vi "EventLog.Filter.vi"(0 "data in":T3[](array[typedef]) {"ts" format="%<%X\n%x>T"}, 1 "Event.Sets":T1 {"Source" items=["Scanner Prod"]; "Level" items=["Warning"]; "dtm_End" format="%<%.1X\n%x>T"; "dtm_Begin" format="%<%.1X\n%x>T"}) -> (2 "data out":T3[](array[typedef]) {"ts" format="%<%X\n%x>T"})   [LabVIEW 2016]
uses:
  EventLog.EventGui.ctl
  EventLog.EventLevel.ctl
  EventLog.EventSource.ctl
  Translator/Translator.Message.ctl
  EventLog.Gui.Sets.ctl
  EventLog.EventLevelOperatorGui.ctl
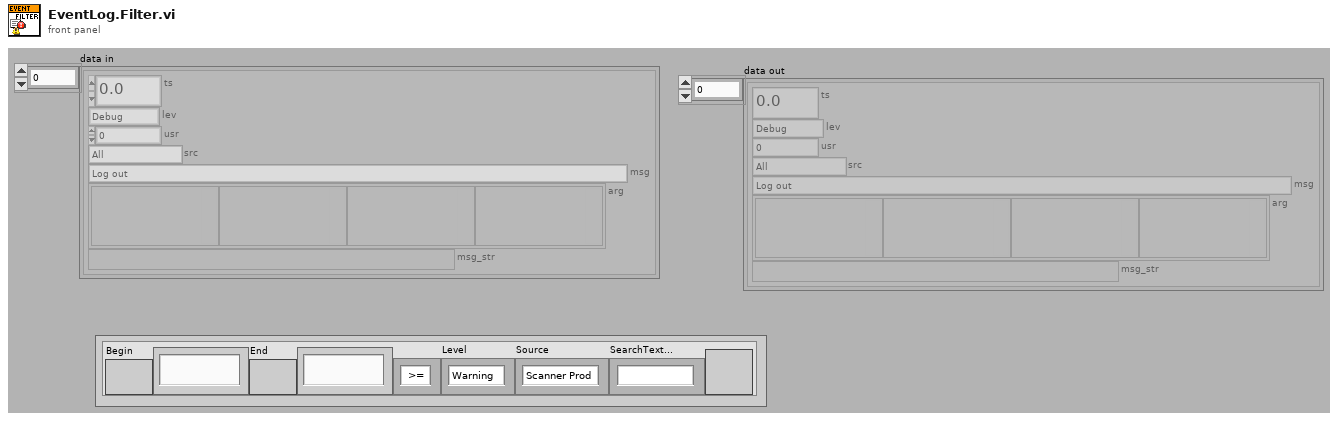
[diagram p1: front panel]
types:
  T1 = typedef "EventLog.Gui.Sets.ctl" = cluster{"IncludeBegin":bool, "dtm_Begin":timestamp, "IncludeEnd":bool, "dtm_End":timestamp, "Events Level Operator":T2, "Level":u16, "Source":u16, "SearchText":string, "Freeze":bool}
  T2 = typedef "EventLog.EventLevelOperatorGui.ctl" = enum16{">=", "=", "<="}
  T3 = typedef "EventLog.EventGui.ctl" = cluster{"ts":dbl, "lev":T4, "usr":i32, "src":T5, "msg":T6, "arg":variant[], "msg_str":string}
  T4 = typedef "EventLog.EventLevel.ctl" = enum8{"Debug", "Info", "Warning", "Error"}
  T5 = typedef "EventLog.EventSource.ctl" = enum16{"All", "Gui", "Ref", "File", "Arch", "Seq", "CPX", "DB", "Laser", "Scan.P", "Scan.O"}
  T6 = typedef "Translator.Message.ctl" = enum16{"-", "Event confirmed", "Log out", "Log in", "Shutdown", "Cancel", "Start", "Begin time", "End time", "Duration", "Service Mode", "Ignore Results", "Serial Format", "On", "Off", "OK", "NOK", "NOK %s", "Home", "Work", "Close", "Open", "In progress...", "Missing", "Empty", "Hardware failure", "Initial", "Default", "Total", "Out of range", "Free disk space is below 1GB - contact technician", "Error %d >> %s", "Error %d >> %s >> %s", "Msg %d >> %s", "Laser msg %d %s", "Laser cmd error %s %d", "Laser cmd failed %s", "Laser cmd warning %s", "Laser disconnected", "Laser status %s", "Laser already started", "Laser job unkonwn %s", "Laser job missing %s", "Laser job select failure %s", "Unable to start laser printing (%s)", "Unable to stop laser printing (%s)", "Laser marking aborted", "Laser marking timeout", "Unable to reset Laser Interlock (%s)", "Unable to trigger Laser. Laser not ready (%s)", "Laser job '%s' coordinates not configured", "Starting %s", "Quitting %s", "Configured", "Initializing", "Quitting", "Loading", "Loaded %d results", "Loaded %d events", "Running", "Stopped", "Summary", "Laser", "Do you want to continue?", "Do you want to delete the configuration?", "The configuration is being used by an order. Unable to delete!", "Press confirm button", "Station is not based. Do you want to exit?", "Station requires changeover. Do you want to run the test?", "Test options are not set as default. Do you want to continue?", "Formatting of WabcoNo is disabled. Do you want to continue?", "Product not detected. Do you want to continue?", "Product scan failed. Do you want to continue?", "Calibration", "Log out?", "System", "All", "IDLE", "Translating...%s", "Not found", "Alarm %s", "Run", "Skip", "Abort", "Repeat", "Please wait...", "Database disconnected", "Database disconnected - changeover disabled!", "Login to database successful", "Login to database failed: %d; %s", "Unable to check the product status of reference %d - database disconnected", "Unable to set the product status of reference %d - database disconnected", "Variant file backup %s", "Read variant (%s)", "Result", "Station armed!", "Station requires changeover!", "Select reference number...", "EMERGENCY BUTTON - press Control button", "EMERGENCY DOOR - press Control button", "Resetting Emergency...", "Unable to reset safety circuit - Emergency Button pressed", "Unable to reset safety circuit - Emergency Side Door open", "Station not based", "Station based", "Station not empty", "Station basing...", "No order", "Press Start to begin new order", "Scanning new order", "Order NOK. Correct or scan again", "Order OK. Press Accept", "Order ready", "Revolver incorrect", "Fork incorrect", "Revolver missing", "Revolver empty", "Container missing", "Offline results", "Offline statistics", "Updating statistics %.1f %%", "DMC Configurator", "Door open", "Close the front door", "Press start button", "Done. Open the front door", "Running...", "Running...%.1f %%", "Pause %s", "Pause %s. NOK container missing", "Pause %s. OK container missing", "Pause %s. Revolver empty", "Pause %s. Revolver missing", "Pause %s. Revolver incorrect", "Pause %s. Fork missing", "Pause %s. Fork incorrect", "Pause %s. Too many failures", "Pause %s. Unloading failure", "Pause %s. One slot is not working", "Pause %s. Part order is done. Empty OK container", "Pause %s. Unable to move product to slot", "Pause %s. Unable to move back product pusher", "Pause %s. Unable to lift product", "Pause %s. Unable to move back product lifter", "Pause %s. Unable to move product arm to Work", "Pause %s. Unable to move product arm to NOK", "Pause %s. Unable to move product arm to OK", "Pause %s. Unable to unsuck the NOK product", "Pause %s. Unable to drop the NOK product", "Pause %s. Product OK missing", "Pause %s. Unable to unsuck the OK product", "Pause %s. Unable to drop the OK product", "Stopping...", "File '%s' is missing", "File '%s' is broken", "File '%s' is running", "Log file started (%s)", "Log file ended (%s)", "Log file stopped (%s)", "Log file ignored (%s)", "Log file exported (%s)", "Log file export failed (%s)", "Wrong serial number in log file", "Wrong reference number in log file", "Test steps are missing", "%s = %.3f", "Process param '%s' not found in DB", "Process param '%s' wrong order", "Process param '%s' value %.3f out of limits (%.3f; %.3f)", "Step%d param '%s' not found in DB", "Step%d param '%s' wrong order", "Step%d param '%s' value %.3f out of limits (%.3f; %.3f)", "Step%d EV '%s' not found in DB", "Step%d EV '%s' wrong order", "\"%s\" not found in DB", "\"%s\" wrong order", "\"%s\" value %.3f out of limits (%.3f; %.3f)", "\"%s\" not found in software", "Process init (%s)", "Process started", "Process restarted", "Process run", "Process done", "Process done - remove OK container", "Process aborted", "Process aborted at work", "Process aborted at home", "Process error", "Process error at home", "Process error at work", "Process close", "Process pause", "Process continue", "Process door open", "Process door close", "Process pause at slot %s due to %s", "Select plate from the order to process", "Do you want to start the process?", "Do you want to continue the process?", "There is unfinished order. Do you want to put the new order?", "Product %s %d OK", "Product %s %d NOK", "Unable to unload the slot %s. Product missing in the slot", "Unable to unload the slot %s. Product already in the arm", "Unable to accept the product as OK. Product missing in slot %s", "Unable to accept the product as OK. Product could not drop into the container at slot %s", "Unable to accept the product as NOK. Product could not drop into the container at slot %s", "Scan failed. Error %s", "Scan failed. Scanner disconnected", "Scan failed. Wrong Wabco number %d, limit (%d,%d)", "Scan failed. Wrong serial number %d, limit (%d,%d)", "Scan failed. Wrong date %d, limit (%d,%d)", "Scan failed. Wrong product wabco number %d (expected %d)", "Scan failed. Wrong product serial number %d (expected > 0)", "Scan OK %s", "Scan failed. Unable to determine table position (%s)", "Scan failed. Timeout", "Tune failed. Scanner disconnected", "Tune failed. Timeout", "%s = %d", "%s = %d->%d", "Unable to set %s = %.2f - Air Pressure Inside off", "Unable to set digital output '%s' = %d", "Unable to activate air pressure inside - timeout", "Unable to activate air pressure inside - aborted", "Unable to switch on Air Main Valve - Air Pressure Inlet off", "Unable to switch on Air Main Valve - Door open", "Unable to switch off Air Main Valve - timeout", "Unable to switch off Air Main Valve - aborted", "Unable to rotate Table - timeout", "Unable to rotate Table - aborted", "Unable to rotate Table - Product Move not in Home position", "Unable to rotate Table - Air Pressure Inside off", "Unable to rotate Table - Product Lift A not in Home position", "Unable to rotate Table - Product Lift B not in Home position", "Unable to rotate Table - unlock before movement timeout", "Unable to rotate Table - lock after movement timeout", "Unable to move Table Lock to %s position - timeout", "Unable to move Table Lock to %s position - aborted", "Unable to move Table Lock to %s position - Air Pressure Inside off", "Unable to move Table Lock to %s position - Table not in position", "Unable to move Product Lift A to %s position - timeout", "Unable to move Product Lift B to %s position - timeout", "Unable to move Product Lift A to %s position - aborted", "Unable to move Product Lift B to %s position - aborted", "Unable to move Product Lift A to %s position - Air Pressure Inside off", "Unable to move Product Lift B to %s position - Air Pressure Inside off", "Unable to move Product Lift A to %s position - Table not locked", "Unable to move Product Lift B to %s position - Table not locked", "Unable to move Product Lift A to %s position - Product Arm not in Work position", "Unable to move Product Lift B to %s position - Product Arm not in Work position", "Unable to set Product Suction Gripper %s to %s - timeout", "Unable to set Product Suction Gripper %s to %s - aborted", "Unable to set Product Suction Gripper %s to %s - Air Pressure Inside off", "Unable to set Product Suction Gripper %s to %s - Table slot unkown", "Unable to move Product Arm to %s position - timeout", "Unable to move Product Arm to %s position - aborted", "Unable to move Product Arm to %s position - Air Pressure Inside off", "Unable to move Product Arm to %s position - Product Lift A not in Home position", "Unable to move Product Arm to %s position - Product Lift B not in Home position", "Unable to move Product to %s position - timeout", "Unable to move Product to %s position - aborted", "Unable to move Product to %s position - Air Pressure Inside off", "Unable to move Product to %s position - Table not in position"}
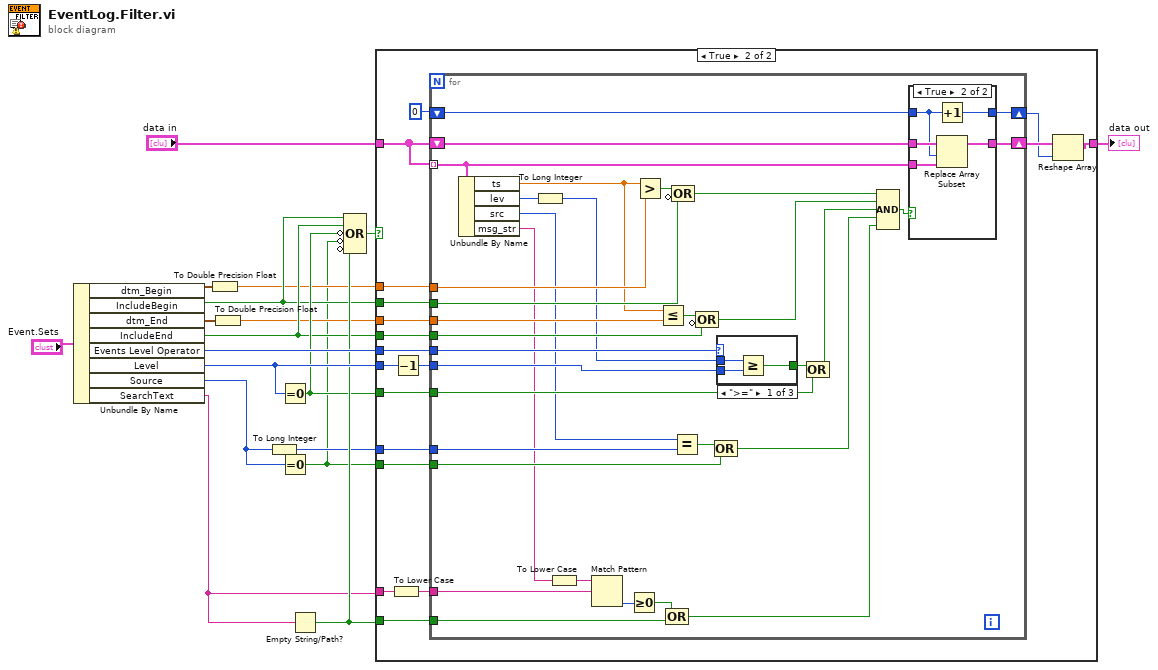
[diagram p0: block diagram]
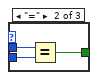
[diagram p4: hidden frame]
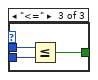
[diagram p5: hidden frame]
diagram:
  n1 = Unbundle By Name("Event.Sets") -> ("dtm_Begin"=w18:timestamp, "IncludeBegin"=w9:bool, "dtm_End"=w17:timestamp, "IncludeEnd"=w10:bool, "Events Level Operator"=w16:T2, "Level"=w13:u16, "Source"=w2:u16, "SearchText"=w7:string)
  n2 = To Double Precision Float(number=w18) -> (double precision float=w5:dbl)
  n3 = To Double Precision Float(number=w17) -> (double precision float=w4:dbl)
  n4 = To Long Integer(number=w2) -> (32bit integer=w3:i32)
  n5 = Equal To 0?(x=w13) -> (x = 0?=w11:bool)
  n6 = Equal To 0?(x=w2) -> (x = 0?=w1:bool)
  n7 = Empty String/Path?(string/path=w7) -> (empty?=w12:bool)
  n8 = Compound Arithmetic op=OR(w9, w10, invert w11, invert w1, invert w12) -> (w8:bool)
  n9 = case shown="True" w8 {
    tunnel: w5 -> [_ w37]
    tunnel: w9 -> [_ w36]
    tunnel: w4 -> [_ w35]
    tunnel: w10 -> [_ w34]
    tunnel: w16 -> [_ w33]
    tunnel: w11 -> [_ w32]
    tunnel: [w19 w28] -> w15
    tunnel: "data in" -> [w19 w27]
    tunnel: w13 -> [_ w26]
    tunnel: w7 -> [_ w24]
    tunnel: w12 -> [_ w23]
    tunnel: w3 -> [_ w20]
    tunnel: w1 -> [_ w21]
    frame False {
    }
    frame True {
      n10 = To Lower Case(string=w24) -> (all lower case string=w25:string)
      n11 = Decrement(x=w26) -> (x-1=w22:u16)
      n12 = for {
        tunnel: w27 -> [w38] mode=indexing
        tunnel: w37 -> [w71]
        tunnel: w36 -> [w70]
        tunnel: w35 -> [w68]
        tunnel: w34 -> [w66]
        tunnel: w33 -> [w64]
        tunnel: w22 -> [w61]
        tunnel: w32 -> [w62]
        shift-right: [w55] -> w30
        shift-left: w27 -> [w56]
        shift-right: [w52] -> w29
        shift-left: 0 -> [w53]
        tunnel: w25 -> [w51]
        tunnel: w23 -> [w47]
        tunnel: w20 -> [w43]
        tunnel: w21 -> [w44]
        n13 = Unbundle By Name(w38) -> ("ts"=w65:dbl, "lev"=w63:T4, "src"=w41:T5, "msg_str"=w42:string)
        n14 = To Long Integer(number=w63) -> (32bit integer=w60:i32)
        n15 = To Lower Case(string=w42) -> (all lower case string=w46:string)
        n16 = Match Pattern(string=w46, regular expression=w51) -> (offset past match=w49:i32)  [unwired: 1 in, 3 out]
        n17 = Greater Or Equal To 0?(x=w49) -> (x >= 0?=w48:bool)
        n18 = Greater?(x=w65, y=w71) -> (0:w69:bool)
        n19 = Less Or Equal?(x=w65, y=w68) -> (x <= y?=w67:bool)
        n20 = Compound Arithmetic op=OR(w48, w47) -> (w50:bool)
        n21 = Compound Arithmetic op=OR(w69, invert w70) -> (w57:bool)
        n22 = Equal?(x=w41, y=w43) -> (x = y?=w40:bool)
        n23 = Compound Arithmetic op=OR(w67, invert w66) -> (w58:bool)
        n24 = Compound Arithmetic op=OR(w40, w44) -> (w39:bool)
        n25 = case shown="\">=\"" w64 {
          tunnel: w60 -> [w81 w84 w87]
          tunnel: w61 -> [w80 w83 w86]
          tunnel: [w79 w82 w85] -> w59
          frame ">=" {
            n26 = Greater Or Equal?(x=w81, y=w80) -> (x >= y?=w79:bool)
          }
          frame "=" {
            n27 = Equal?(x=w84, y=w83) -> (x = y?=w82:bool)
          }
          frame "<=" {
            n28 = Less Or Equal?(x=w87, y=w86) -> (x <= y?=w85:bool)
          }
        }
        n29 = Compound Arithmetic op=OR(w59, w62) -> (w45:bool)
        n30 = Compound Arithmetic op=AND(w57, w58, w45, w39, w50) -> (w54:bool)
        n31 = case shown="True" w54 {
          tunnel: w56 -> [w73 w78]
          tunnel: [w73 w77] -> w55
          tunnel: w38 -> [_ w76]
          tunnel: w53 -> [w72 w75]
          tunnel: [w72 w74] -> w52
          frame False {
          }
          frame True {
            n32 = Increment(x=w75) -> (x+1=w74:i32)
            n33 = Replace Array Subset(array=w78, new element=w76, index=w75) -> (w77:T3[])
          }
        }
      }
      n34 = Reshape Array(w30, w29) -> (w28:T3[])
    }
  }
  "data out" <- w15
